vi "Get Name.vi"(8 "error in (no error)":errorcluster, 11 "Dependency Source in":refnum<class "Dependency Source.lvclass">) -> (0 "error out":errorcluster, 2 "Dependency Source Name":string, 3 "Dependency Source out":refnum<class "Dependency Source.lvclass">)   [LabVIEW 2019, in "Project.Dependencies Finder.lvlib" / "Dependency Source.lvclass"]
doc: "Return the name of the dependency source. \n\nOnly non-empty strings are valid."
uses:
  Dependency Source.lvclass
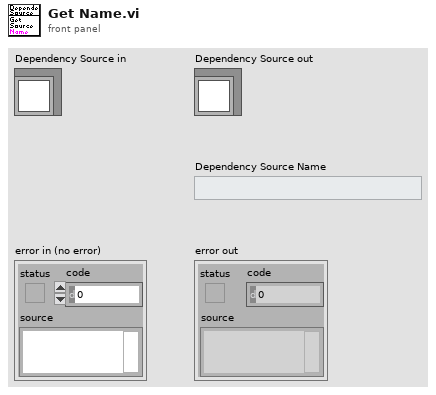
[diagram p1: front panel]
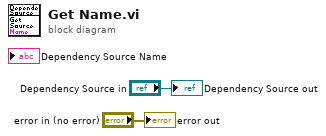
[diagram p0: block diagram]
diagram:
  "error out" <- "error in (no error)"
  "Dependency Source out" <- "Dependency Source in"
